vi "Get Character.vi"(11 "string":string) -> (3 "image data":T1)   [LabVIEW 2021, in "Picture Pixel Fonts.lvlib" / "Pixel Font.lvlib"]
uses:
  Pixel Font.lvlib
  <vilib>/picture/picture.llb/imagedata.ctl
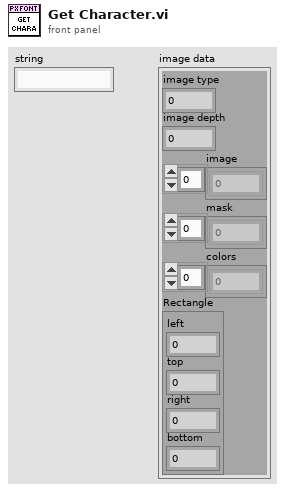
[diagram p1: front panel]
types:
  T1 = typedef "imagedata.ctl" = cluster{"image type":i32, "image depth":i32, "image":u8[], "mask":u8[], "colors":u32[], "Rectangle":cluster{"left":i16, "top":i16, "right":i16, "bottom":i16}}
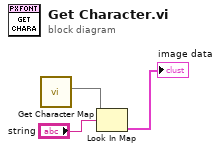
[diagram p0: block diagram]
diagram:
  n1 = call "Get Character Map.vi"() -> ("Symbol Map (Small Fonts 8)"=w1:map{string, T1})  [unwired: 11 in]
  n2 = Look In Map(map=w1, key="string") -> (value=→"image data":T1)  [unwired: 1 in, 1 out]
